vi "Time_ElapsedTime.vi"(9 "PassthroughTime_SEC":dbl=-1.0, 11 "Reset":bool) -> (3 "Elapsed Time Sec":dbl)   [LabVIEW 2019, in "Trajectory_Library.lvlib"]
doc: "This function retruns the number of seconds that have passed since the RESET input has been true. If RESET has never been true then the time since the first call to this routine is returned.\n\nInputs:\n -- Reset -- boolean -- Restart the elapsed time. This remembers the current time.\n -- PassthroughTime -- double float -- Elapsed time clock. (Optional. Default: Read FPGA clock)\n\nOutputs:\n -- Elapsed Time -- double -- Number of seconds that have passed since the reset input was TRUE."
uses:
  Util_GetTime_U32.vi
  Util_GetTime_U64.vi
  Trajectory_Library.lvlib
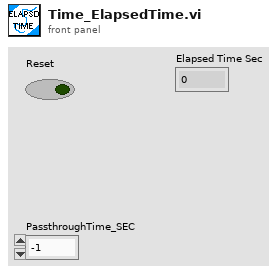
[diagram p1: front panel]
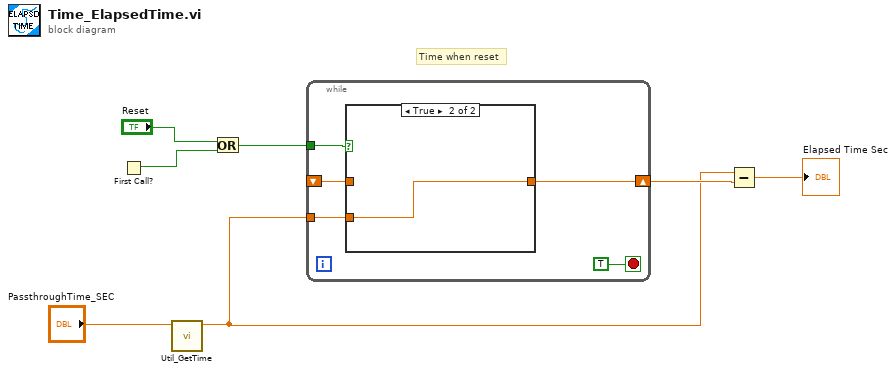
[diagram p0: block diagram]
diagram:
  # "Time when reset"
  n1 = First Call?() -> (First Call?: T/F=w5:bool)
  n2 = call "Util_GetTime.vi"("Pass_Through_Time"="PassthroughTime_SEC") -> ("FPGA_Time_Seconds"=w2:dbl)  [unwired: 8 in, 2 out]
  n3 = Or(x="Reset", y=w5) -> (x .or. y?=w4:bool)
  n4 = while {
    tunnel: w2 -> [w10]
    tunnel: w4 -> [w11]
    shift-right: [w9] -> w3
    shift-left: _ -> [w8]
    stop <- TRUE stop-if-true
    n5 = case shown="True" w11 {
      tunnel: w10 -> [_ w14]
      tunnel: [w13 w14] -> w9
      tunnel: w8 -> [w13 _]
      frame False {
      }
      frame True {
      }
    }
  }
  n6 = Subtract(x=w2, y=w3) -> (x-y=→"Elapsed Time Sec":dbl)
